vi "open_Script_Window_dyn.vi"(4 "AnalysisData":string[](array[string]), 6 "AnalysisSessionID":string, 8 "error in (no error)":errorcluster, 9 "run/stop button":bool, 10 "Script Path":path) -> (0 "error out":errorcluster)   [LabVIEW 2018]
doc: "opens/starts the Script window dynamically"
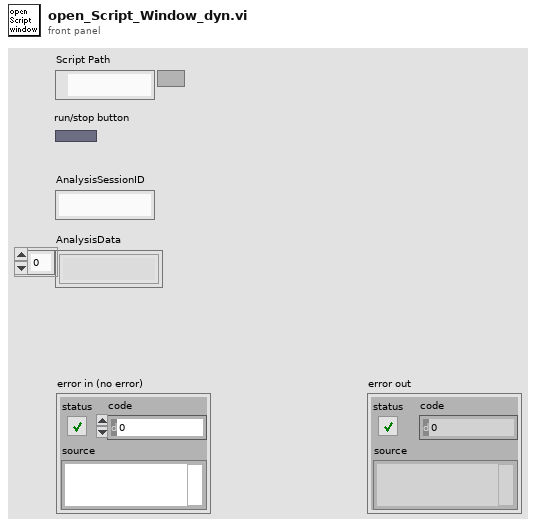
[diagram p1: front panel]
types:
  T1 = enum32{"Invalid", "Standard", "Closed", "Hidden", "Minimized", "Maximized"}
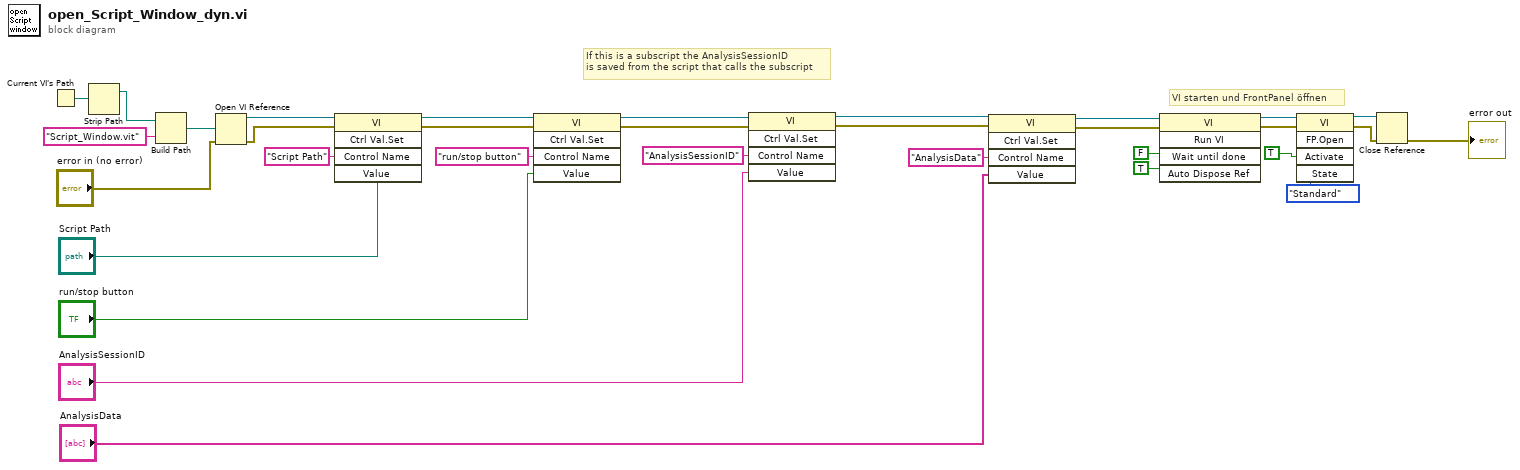
[diagram p0: block diagram]
diagram:
  # "If this is a subscript the AnalysisSessionID\nis saved from the script that calls the subscript"
  # "VI starten und FrontPanel öffnen"
  n1 = Current VI's Path() -> (path=w12:path)
  n2 = Strip Path(path=w12) -> (stripped path=w11:path)  [unwired: 1 out]
  n3 = Build Path(base path=w11, name or relative path="Script_Window.vit") -> (appended path=w24:path)
  n4 = Open VI Reference(vi path=w24, error in (no error)="error in (no error)") -> (vi reference=w22:refnum<vi>, error out=w21:errorcluster)  [unwired: 4 in]
  n5 = invoke class="VI" method="Ctrl Val.Set"(reference=w22, error in=w21, "Control Name"="Script Path", "Value"="Script Path") -> (reference out=w15:refnum<vi>, error out=w14:errorcluster)  [unwired: 1 in, 3 out]
  n6 = invoke class="VI" method="Ctrl Val.Set"(reference=w15, error in=w14, "Control Name"="run/stop button", "Value"="run/stop button") -> (reference out=w9:refnum<vi>, error out=w8:errorcluster)  [unwired: 1 in, 3 out]
  n7 = invoke class="VI" method="Ctrl Val.Set"(reference=w9, error in=w8, "Control Name"="AnalysisSessionID", "Value"="AnalysisSessionID") -> (reference out=w5:refnum<vi>, error out=w4:errorcluster)  [unwired: 1 in, 3 out]
  n8 = invoke class="VI" method="Ctrl Val.Set"(reference=w5, error in=w4, "Control Name"="AnalysisData", "Value"="AnalysisData") -> (reference out=w3:refnum<vi>, error out=w2:errorcluster)  [unwired: 1 in, 3 out]
  n9 = invoke class="VI" method="Run VI"(reference=w3, error in=w2, "Wait until done"=FALSE, "Auto Dispose Ref"=TRUE) -> (reference out=w30:refnum<vi>, error out=w29:errorcluster)  [unwired: 1 in, 3 out]
  n10 = invoke class="VI" method="FP.Open"(reference=w30, error in=w29, "Activate"=TRUE, "State"=T1."Standard") -> (reference out=w26:refnum<vi>, error out=w25:errorcluster)  [unwired: 1 in, 3 out]
  n11 = Close Reference(reference=w26, error in (no error)=w25) -> (error out=→"error out":errorcluster)
